vi "ReadGFGandWriteALLtoINI.vi"(8 "error in (no error)":errorcluster, 10 "exclusion regexp array":string[](array[string]), 11 "Path":path) -> (0 "error out":errorcluster)   [LabVIEW 2012]
doc: "SciScan 1.2 160622\nThis VI reads an INI file and stores all keys in a Generalized Functional Global Variable (GFG). It then monitors updates to the GFG and writes keys back into INI file before closing. Note that the INI file only supports data type DBL or STRING. The GFG can handle any arbitrary data type, but values that are not DBL or STRING are discarded when closing and not written to INI file."
uses:
  <vilib>/Utility/config.llb/Write Key (Double).vi
  <vilib>/Utility/config.llb/Write Key (String).vi
  <vilib>/Utility/config.llb/Write Key (Boolean).vi
  <vilib>/Utility/config.llb/NI_LVConfig.lvlib
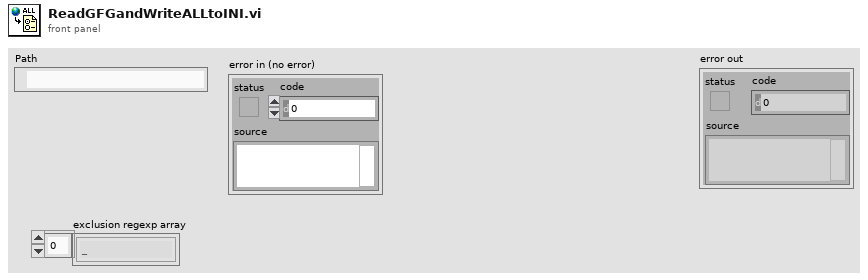
[diagram p1: front panel]
types:
  T1 = typedef "NI_LVConfig.lvlib/Config Data RefNum.ctl" = refnum<k1>
  T2 = typedef "VariantType.lvlib/Type.ctl" = enum8{"Invalid Type", "Void", "I8", "I16", "I32", "I64", "U8", "U16", "U32", "U64", "Single Float", "Double Float", "Extended Float", "Single Complex", "Double Complex", "Extended Complex", "Enum U8", "Enum U16", "Enum U32", "Enum U64", "Single Float With Unit", "Double Float With Unit", "Extended Float With Unit", "Single Complex with Unit", "Double Complex with Unit", "Extended Complex with Unit", "Boolean", "String", "Path", "Picture", "Tag", "Array", "Cluster", "Variant", "LV Variant", "Waveform", "Timestamp", "Digital Waveform", "Digital Data", "ExpressData", "Refnum", "External Data", "VI", "Poly VI", "LabVIEW Class Instance", "Fixed Point"}
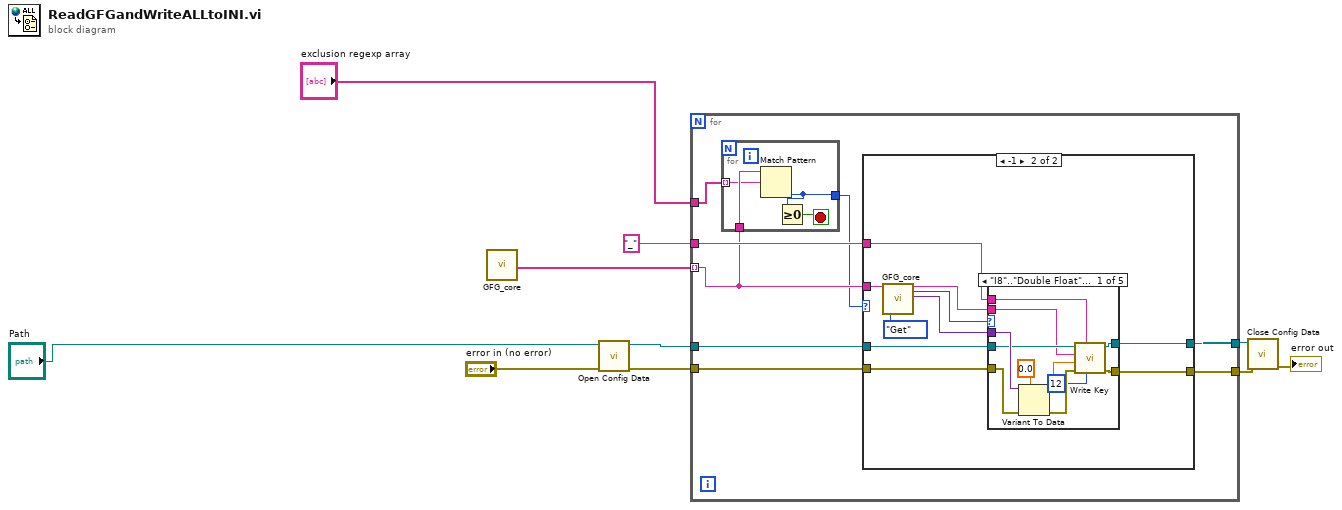
[diagram p0: block diagram]
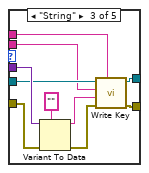
[diagram p4: hidden frame]
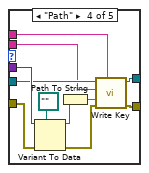
[diagram p5: hidden frame]
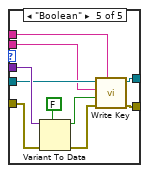
[diagram p6: hidden frame]
diagram:
  n1 = call "GFG_core.vi"() -> ("All Variable Names Out"=w3:string[])  [unwired: 13 in, 6 out]
  n2 = call <vilib>:"Open Config Data.vi"("error in (no error)"="error in (no error)", "configuration file path"="Path") -> ("error out"=w8:errorcluster, "refnum"=w9:T1)  [unwired: 7 in, 1 out]
  n3 = for {
    tunnel: [w17] -> w5
    tunnel: w9 -> [w16]
    tunnel: w8 -> [w18]
    tunnel: [w15] -> w6
    tunnel: w3 -> [w13] mode=indexing
    tunnel: "_" ("Variable Name") -> [w14]
    tunnel: "exclusion regexp array" -> [w12]
    n4 = for {
      tunnel: w13 -> [w22]
      tunnel: w12 -> [w21] mode=indexing
      tunnel: [w19] -> w11
      stop <- w20 stop-if-true
      n5 = Match Pattern(string=w22, regular expression=w21) -> (offset past match=w19:i32)  [unwired: 1 in, 3 out]
      n6 = Greater Or Equal To 0?(x=w19) -> (x >= 0?=w20:bool)
    }
    n7 = case shown="-1" w11 {
      tunnel: w18 -> [w23 w31]
      tunnel: [w23 w30] -> w17
      tunnel: w16 -> [w24 w29]
      tunnel: [w24 w28] -> w15
      tunnel: w14 -> [_ w26]
      tunnel: w13 -> [_ w25]
      frame 0, Default {
      }
      frame -1 {
        n8 = call "GFG_core.vi"("Variable Name in"=w25, "Action"=enum16{"Init", "Set", "Get"}."Get") -> ("Variable Name Out"=w27:string, "Data Type Out"=w33:T2, "Variant Out"=w32:variant)  [unwired: 11 in, 4 out]
        n9 = case shown="\"I8\"..\"Double Float\", \"Enum U8\"..\"Enum U64\"" w33 {
          tunnel: w32 -> [w44 _ w57 w68 w78]
          tunnel: [w41 w47 w54 w66 w75] -> w30
          tunnel: w31 -> [w40 w47 w53 w65 w74]
          tunnel: w29 -> [w39 w46 w52 w64 w73]
          tunnel: [w38 w46 w51 w63 w72] -> w28
          tunnel: w27 -> [w37 _ w50 w62 w71]
          tunnel: w26 -> [w36 _ w49 w61 w70]
          frame "I8".."Double Float", "Enum U8".."Enum U64" {
            n10 = Variant To Data(error in=w40, type=0.0, Variant=w44) -> (data=w43:dbl, error out=w42:errorcluster)
            n11 = call-poly <vilib>:"Write Key.vi"("precision (6)"=i16 12, "section"=w36, "error in (no error)"=w42, "value"=w43, "key"=w37, "refnum"=w39) -> ("error out"=w41:errorcluster, "refnum out"=w38:T1)  [unwired: 3 in, 1 out]
          }
          frame Default {
          }
          frame "String" {
            n12 = Variant To Data(error in=w53, type="" ("Variable Name Out"), Variant=w57) -> (data=w56:string, error out=w55:errorcluster)
            n13 = call-poly <vilib>:"Write Key.vi"("section"=w49, "error in (no error)"=w55, "value"=w56, "key"=w50, "refnum"=w52) -> ("error out"=w54:errorcluster, "refnum out"=w51:T1)  [unwired: 4 in, 1 out]
          }
          frame "Path" {
            n14 = Variant To Data(error in=w65, type=path "" ("configuration file path 2"), Variant=w68) -> (data=w58:path, error out=w67:errorcluster)
            n15 = Path To String(path=w58) -> (string=w59:string)
            n16 = call-poly <vilib>:"Write Key.vi"("section"=w61, "error in (no error)"=w67, "value"=w59, "key"=w62, "refnum"=w64) -> ("error out"=w66:errorcluster, "refnum out"=w63:T1)  [unwired: 4 in, 1 out]
          }
          frame "Boolean" {
            n17 = Variant To Data(error in=w74, type=FALSE, Variant=w78) -> (data=w77:bool, error out=w76:errorcluster)
            n18 = call-poly <vilib>:"Write Key.vi"("section"=w70, "error in (no error)"=w76, "value"=w77, "key"=w71, "refnum"=w73) -> ("error out"=w75:errorcluster, "refnum out"=w72:T1)  [unwired: 4 in, 1 out]
          }
        }
      }
    }
  }
  n19 = call <vilib>:"Close Config Data.vi"("error in (no error)"=w5, "refnum"=w6) -> ("error out"=→"error out":errorcluster)  [unwired: 8 in, 1 out]
